vi "Stop Core.vi"(10 "final error code":i32, 11 "Image Acquisition in":refnum<class "Image Acquisition.lvclass">) -> (3 "Image Acquisition out":refnum<class "Image Acquisition.lvclass">)   [LabVIEW 2019, in "Image Acquisition.lvlib" / "Image Acquisition.lvclass"]
doc: "(<B>Filename</B>: Actor Framework.lvlib:Actor.lvclass:Stop Core.vi)\n\nDefines what the actor does before it stops. Use the <B>final error code</B> input to determine whether the actor shut down in response to an error.\n\nBy default, this method does nothing. A descendant class may override it to define behavior, such as shutting down any processes the actor initiated in its override of the Actor Core method."
uses:
  Image Acquisition.lvclass
  <vilib>/ActorFramework/Actor/Actor.lvclass
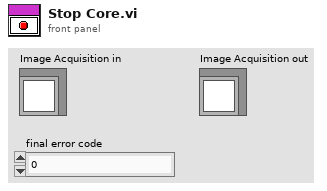
[diagram p1: front panel]
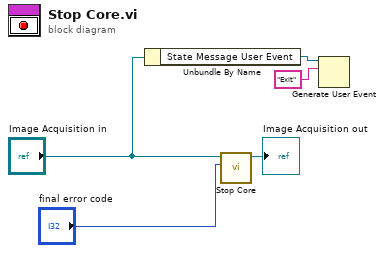
[diagram p0: block diagram]
diagram:
  n1 = Unbundle By Name("Image Acquisition in") -> ("State Message User Event"=w2:refnum<user-event>)
  n2 = call-parent "Stop Core.vi"("final error code"="final error code", "Actor in"="Image Acquisition in") -> ("Actor out"=→"Image Acquisition out":refnum<class "Image Acquisition.lvclass">)  [unwired: 9 in]
  n3 = Generate User Event(user event=w2, event data cluster="Exit" ("event data")) -> ()  [unwired: 2 in, 2 out]
